vi "Test ForLoop Tunnels.vi"() -> ()   [LabVIEW 2018]
panel:
  out "Array":u32[](array[numeric])
  out "tunnels":string[](array[string])
  out "terminals":string[](array[string])
  out "shift regs.":string[](array[string])
  in  "vi path":path=path "C:/Users/lubo/Documents/LabView/LabVIEW-Universal-Transcriptor/Test/Examples For Parsing/Example System Functions.vi"
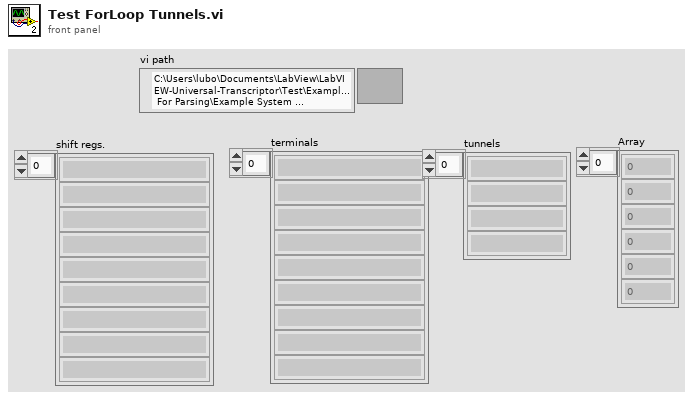
[diagram p1: front panel]
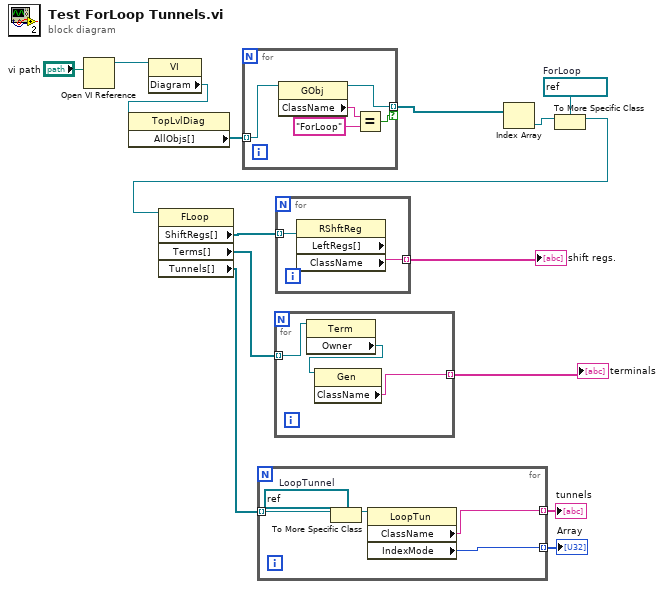
[diagram p0: block diagram]
diagram:
  w9 = refnum<vi> refnum  # ForLoop
  n1 = Open VI Reference(vi path="vi path") -> (vi reference=w14:refnum<vi>)  [unwired: 5 in, 1 out]
  n2 = property class="VI"(reference=w14) -> ("Diagram"=w13:refnum<vi>)  [unwired: 1 in, 2 out]
  n3 = property class="TopLvlDiag"(reference=w13) -> ("AllObjs[]"=w12:refnum<vi>[])  [unwired: 1 in, 2 out]
  n4 = for {
    tunnel: w12 -> [w20] mode=indexing
    tunnel: [w18] -> w11 mode=indexing if=w19
    n5 = property class="GObj"(reference=w20) -> (reference out=w18:refnum<vi>, "ClassName"=w16:string)  [unwired: 1 in, 1 out]
    n6 = Equal?(x=w16, y="ForLoop") -> (x = y?=w19:bool)
  }
  n7 = Index Array(array=w11) -> (element=w10:refnum<vi>)  [unwired: 1 in]
  n8 = To More Specific Class(target class=w9, reference=w10) -> (specific class reference=w8:refnum<vi>)  [unwired: 1 in, 1 out]
  n9 = property class="FLoop"(reference=w8) -> ("ShiftRegs[]"=w7:refnum<vi>[], "Terms[]"=w5:refnum<vi>[], "Tunnels[]"=w3:refnum<vi>[])  [unwired: 1 in, 2 out]
  n10 = for {
    tunnel: w3 -> [w25] mode=indexing
    tunnel: [w22] -> w2 mode=indexing
    tunnel: [w21] -> w1 mode=indexing
    w24 = refnum<vi> refnum  # LoopTunnel
    n11 = To More Specific Class(target class=w24, reference=w25) -> (specific class reference=w23:refnum<vi>)  [unwired: 1 in, 1 out]
    n12 = property class="LoopTun"(reference=w23) -> ("ClassName"=w22:string, "IndexMode"=w21:u32)  [unwired: 1 in, 2 out]
  }
  "tunnels" <- w2
  "Array" <- w1
  n13 = for {
    tunnel: w5 -> [w28] mode=indexing
    tunnel: [w26] -> w4 mode=indexing
    n14 = property class="Term"(reference=w28) -> ("Owner"=w27:refnum<vi>)  [unwired: 1 in, 2 out]
    n15 = property class="Gen"(reference=w27) -> ("ClassName"=w26:string)  [unwired: 1 in, 2 out]
  }
  "terminals" <- w4
  n16 = for {
    tunnel: w7 -> [w30] mode=indexing
    tunnel: [w29] -> w6 mode=indexing
    n17 = property class="RShftReg" props=["LeftRegs[]", "ClassName"](reference=w30) -> ("ClassName"=w29:string)  [unwired: 1 in, 3 out]
  }
  "shift regs." <- w6
